vi "AnalysisConfig.vi"(8 "error in (no error)":errorcluster, 11 "AnalysisConfig":T6={"PortName"="WLAN_DUT0_ANT0", "PhyPort"=enum."Port5", "ExternalAtt"=0, "TriggerLevel"=-40, "NumberofChain"=1, "AcqLength"=0.0001, "MCSIndex"=7.0, "PhyType"=enum."OFDM", "Standard"=enum."802.11 n", "BW"=enum."20M", "TriggerSource"=enum."RIO0", "Freq"=5180000000.0, "LegacyDataRate"=enum."R1M", "PhyPort2"=enum."Port5", "Freq2"=5180000000.0, "ReferenceLevel(Peak)"=0.0}) -> (0 "error out":errorcluster, 3 "AnalysisConfigCMD":string[](array[string])=["MEMory:TABLe:DELete:ALL", "ROUTe:RFSG:PORT:DELete:ALL", "TRIG:RFSA:WLAN:EDGE RISING", "TRIG:RFSA:WLAN:MQTime  5e-6", "ROUTe:RFSA:PORT:DEFine 'wlan_DUT0_ant0','Port0'", "CONF:RFSA:WLAN:CSEG:EATT:ALL 0", "TRIG:RFSA:WLAN:SOUR 'RF0'", "TRIG:RFSA:WLAN:THR 0", "CONF:RFSA:WLAN:NCH 0", "CONF:RFSA:WLAN:CSEG:PORT \"wlan_DUT0_ant0\"", "CONF:RFSA:WLAN:CSEG:FREQ:CENT 5", "CONF:RFSA:WLAN:BWID 0", "CONF:RFSA:WLAN:STAN A", "CONF:RFSA:WLAN:ALENgth 0", "CONF:RFSA:WLAN:PACK:MCS 0", "CONF:RFSA:WLAN:PHY DSSS", "CONF:RFSA:WLAN:ACT:ALL 1", "CONF:RFSA:WLAN:CSEG:POW:AUTO ON", "CONF:RFSA:WLAN:PACK:NSTS 1 ", "CONF:RFSA:WLAN:PACK:GINT LONG", "CONF:RFSA:WLAN:PACK:DMOD ALL", "CONF:RFSA:WLAN:PACK:PAYL:LENGth 1500", "CONF:RFSA:WLAN:MEAS:MOD:ENAB ON", "CONF:RFSA:WLAN:MEAS:MOD:OFDM:EST:COFF ON", "CONF:RFSA:WLAN:MEAS:MOD:OFDM:EST:IMP ON", "CONF:RFSA:WLAN:MEAS:MOD:OFDM:TRAC:AMPL OFF", "CONF:RFSA:WLAN:MEAS:MOD:OFDM:TRAC:CHAN OFF", "CONF:RFSA:WLAN:MEAS:MOD:OFDM:TRAC:TIME ON", "CONF:RFSA:WLAN:MEAS:MOD:OFDM:TRAC:PHAS NONE", "CONF:RFSA:WLAN:MEAS:MOD:AVER:COUN 50", "CONF:RFSA:WLAN:MEAS:MOD:OFDM:MSYM 16", "CONF:RFSA:WLAN:MEAS:SEM:ENAB ON ", "CONF:RFSA:WLAN:MEAS:SEM:AVER:COUN 3", "CONF:RFSA:WLAN:MEAS:SEM:SPAN:AUTO:ENAB ON", "CONF:RFSA:WLAN:MEAS:OBW:ENAB ON", "CONF:RFSA:WLAN:MEAS:OBW:AVER:COUN 3", "CONF:RFSA:WLAN:MEAS:TXP:ENAB ON", "CONF:RFSA:WLAN:MEAS:TXP:AVER:COUN 3"])   [LabVIEW 2015]
uses:
  PhyPort.ctl
  PhyType.ctl
  standard.ctl
  BW.ctl
  LegacyDataRate.ctl
panel:
  out "size(s)":i32
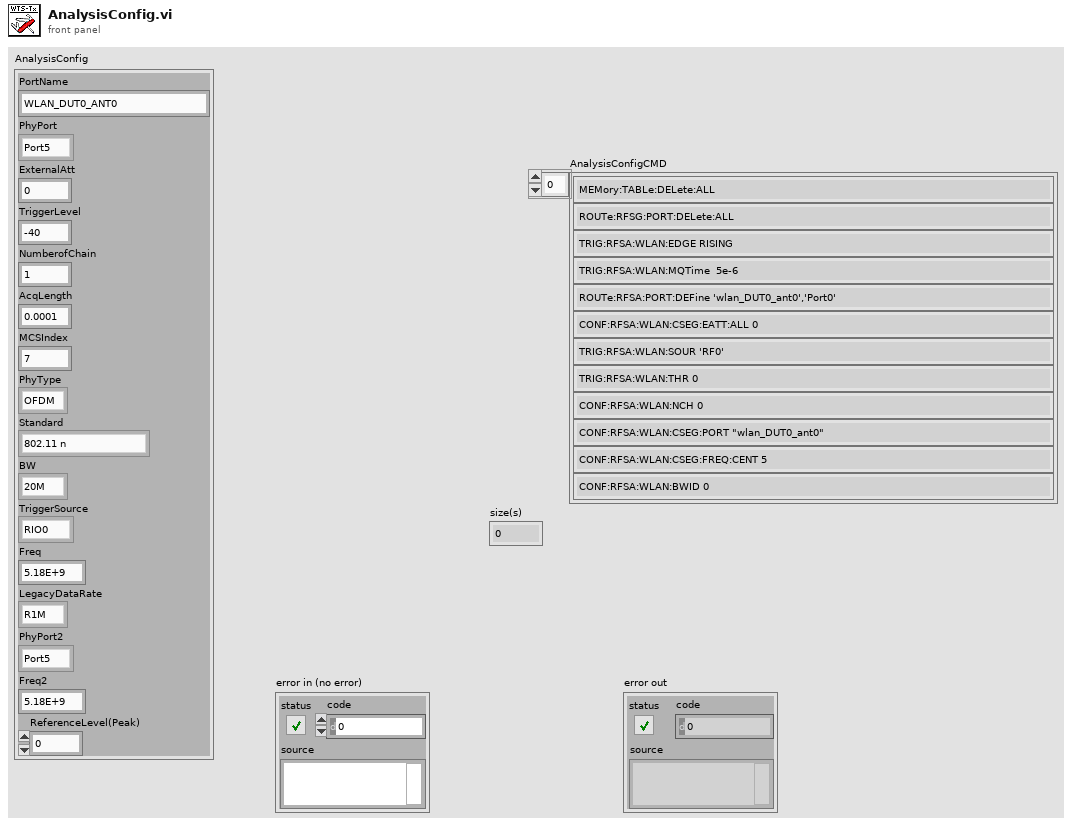
[diagram p1: front panel]
types:
  T1 = typedef "PhyPort.ctl" = enum16{"Port0", "Port1", "Port2", "Port3", "Port4", "Port5", "Port6", "Port7"}
  T2 = typedef "PhyType.ctl" = enum16{"DSSS", "OFDM", "HT", "VHT"}
  T3 = typedef "standard.ctl" = enum16{"802.11 a/g", "802.11 b/g", "802.11 g", "802.11 n", "802.11 ac"}
  T4 = typedef "BW.ctl" = enum16{"5M", "10M", "20M", "40M", "80M", "80P80M", "160M"}
  T5 = typedef "LegacyDataRate.ctl" = enum16{"R1M", "R2M", "R5M5", "R6M", "R9M", "R11M", "R12M", "R18M", "R24M", "R36M", "R48M", "R54M"}
  T6 = cluster{"PortName":string, "PhyPort":T1, "ExternalAtt":i32, "TriggerLevel":i32, "NumberofChain":i32, "AcqLength":dbl, "MCSIndex":dbl, "PhyType":T2, "Standard":T3, "BW":T4, "TriggerSource":enum16{"RIO0", "RIO1"}, "Freq":dbl, "LegacyDataRate":T5, "PhyPort2":T1, "Freq2":dbl, "ReferenceLevel(Peak)":dbl}
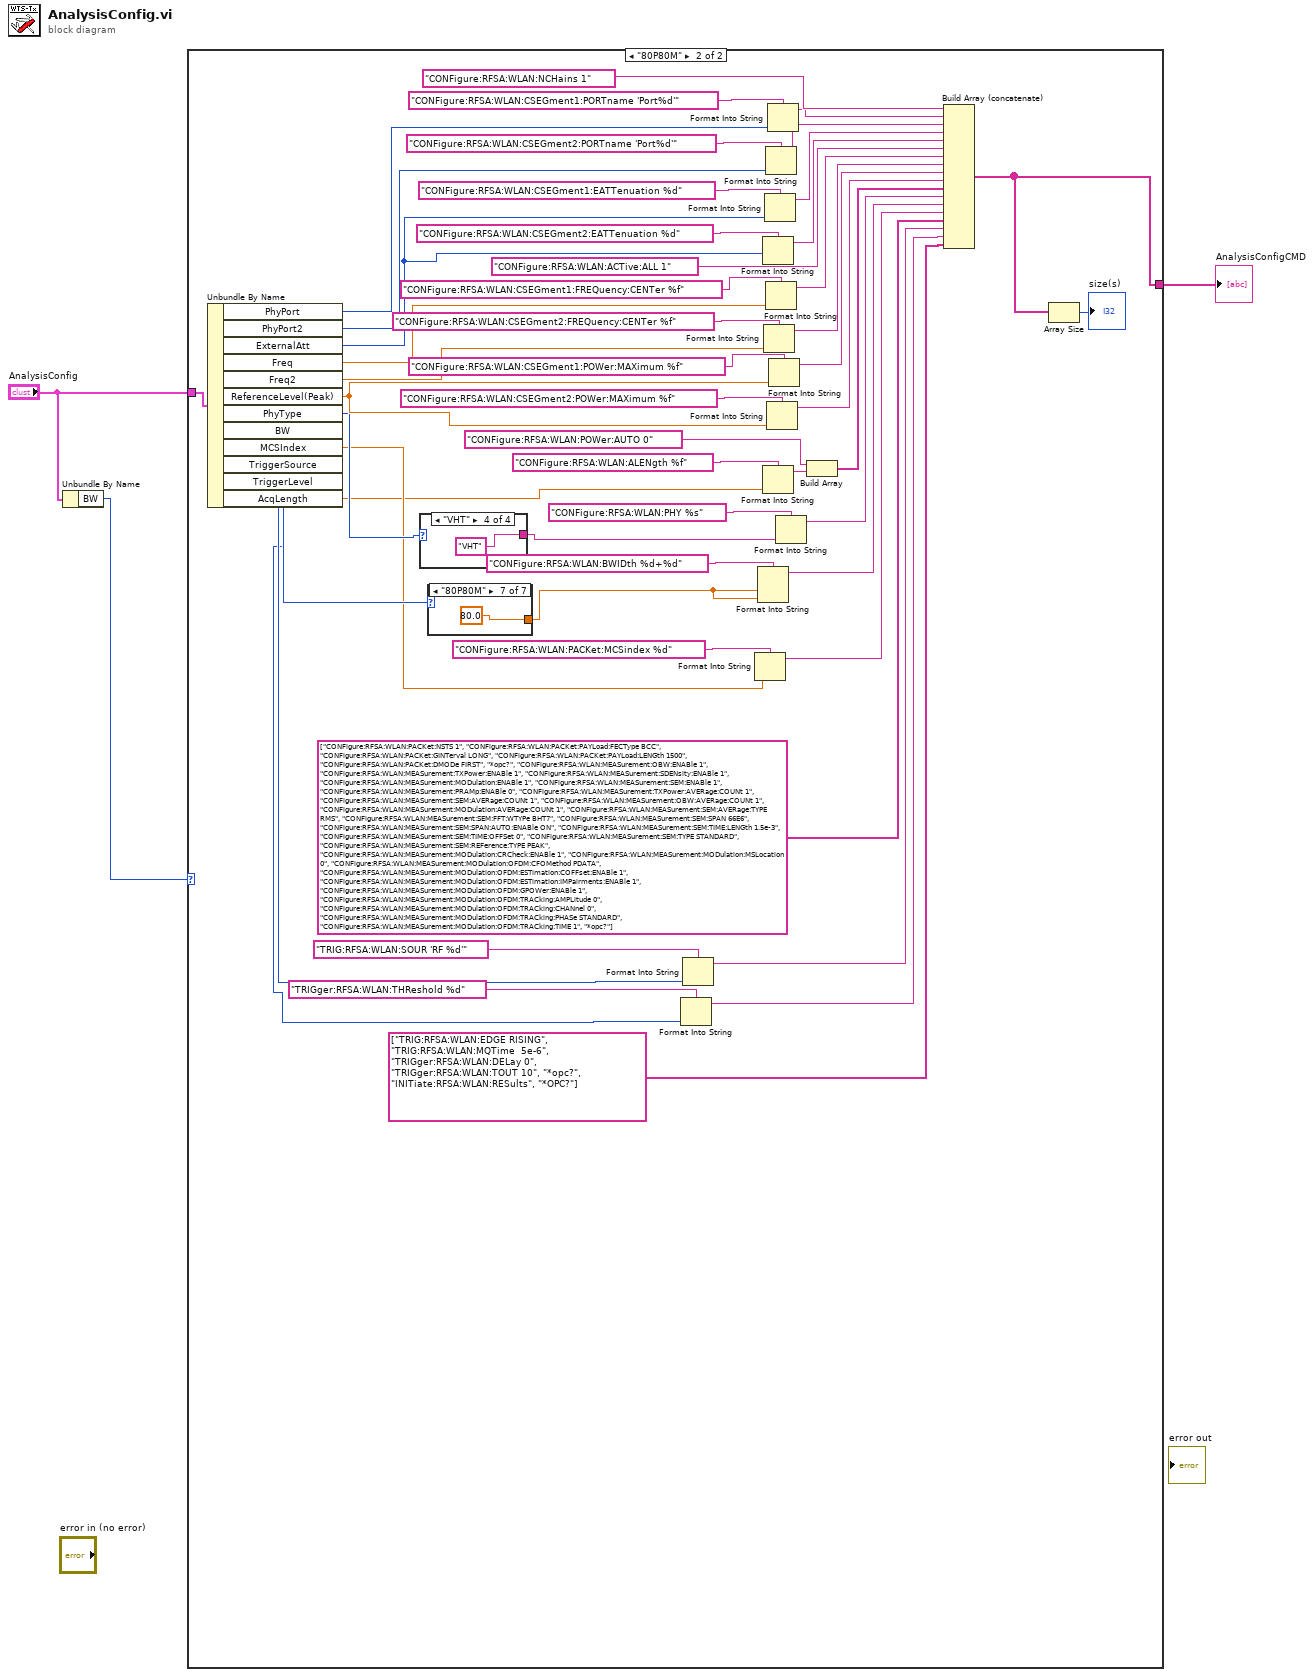
[diagram p0: block diagram]
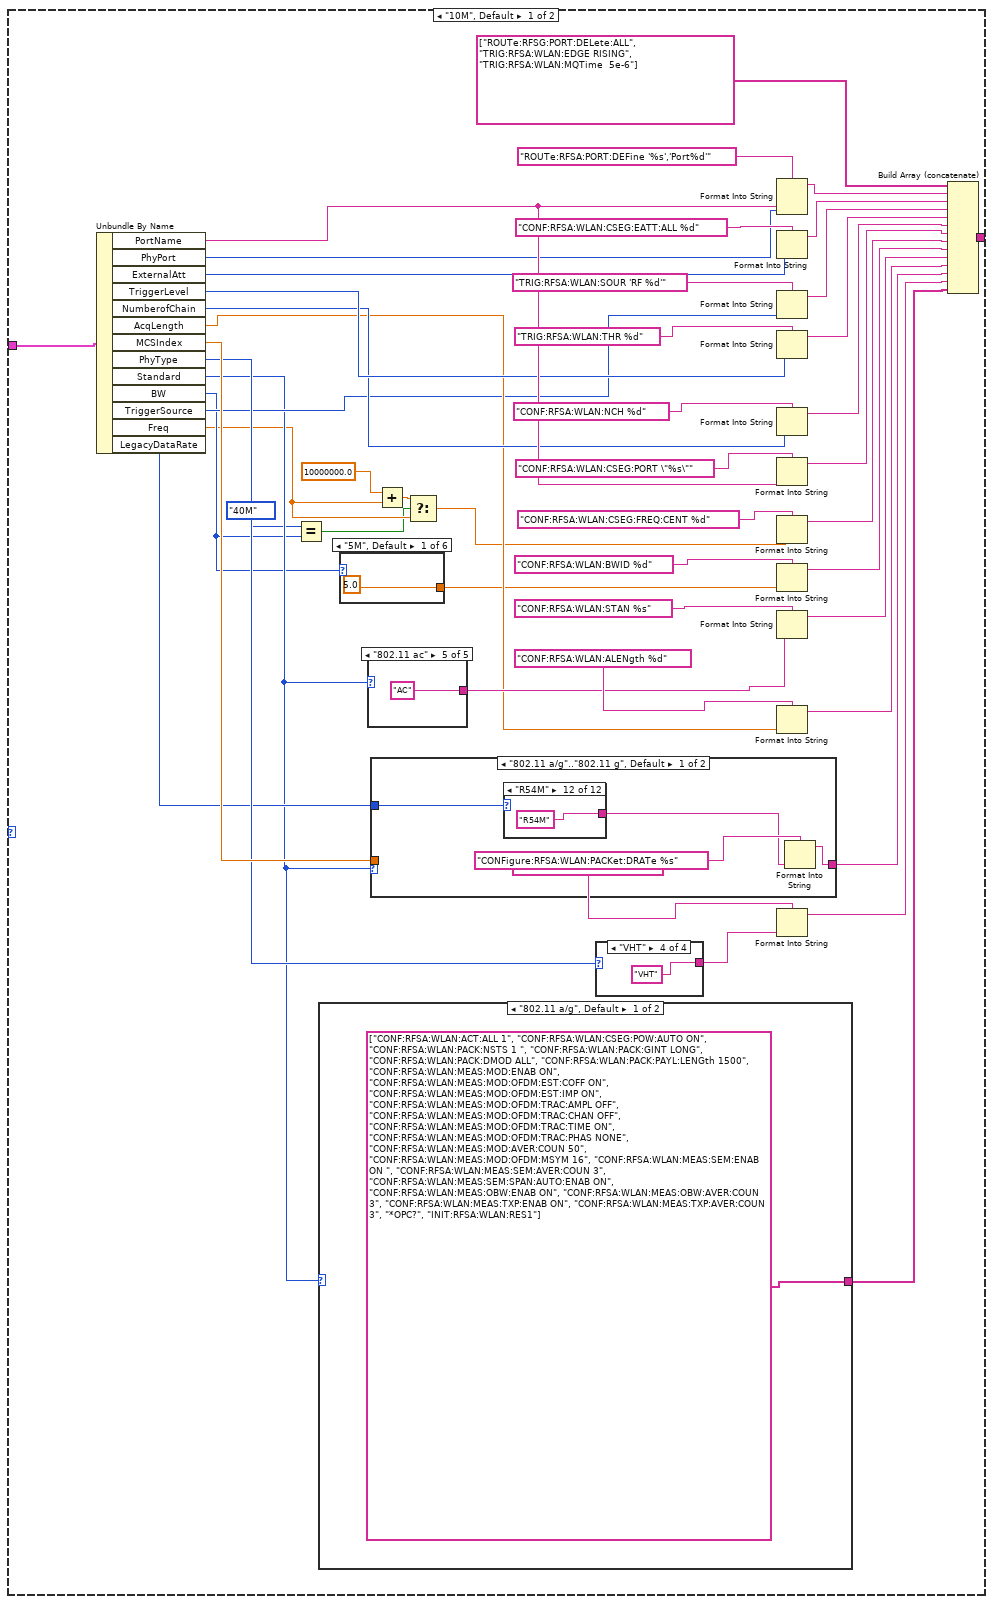
[diagram p2: hidden frame]
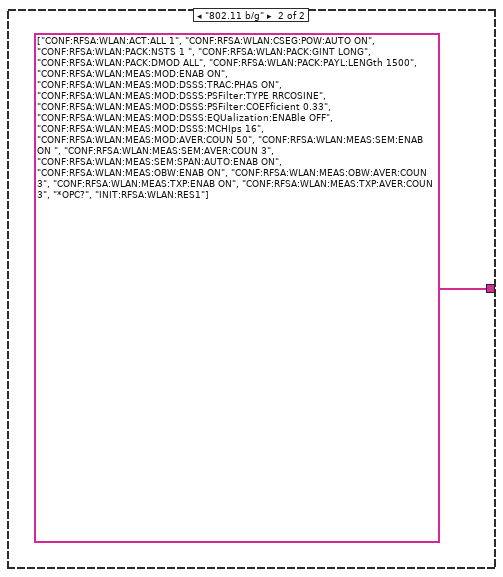
[diagram p3: hidden frame]
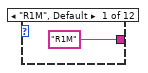
[diagram p4: hidden frame]
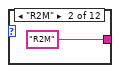
[diagram p5: hidden frame]
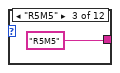
[diagram p6: hidden frame]
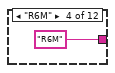
[diagram p7: hidden frame]
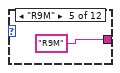
[diagram p8: hidden frame]
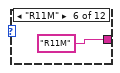
[diagram p9: hidden frame]
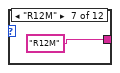
[diagram p10: hidden frame]
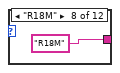
[diagram p11: hidden frame]
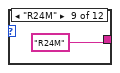
[diagram p12: hidden frame]
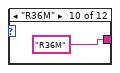
[diagram p13: hidden frame]
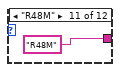
[diagram p14: hidden frame]
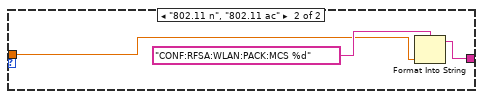
[diagram p15: hidden frame]
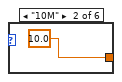
[diagram p16: hidden frame]
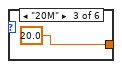
[diagram p17: hidden frame]
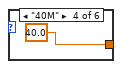
[diagram p18: hidden frame]
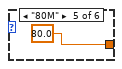
[diagram p19: hidden frame]
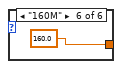
[diagram p20: hidden frame]
diagram:
  n1 = Unbundle By Name("AnalysisConfig") -> ("BW"=w1:T4)
  n2 = case shown="\"80P80M\"" w1 {
    tunnel: [w42 w89] -> w3
    tunnel: "AnalysisConfig" -> [w23 w137]
    frame "10M", Default {
      n3 = Unbundle By Name(w23) -> ("PortName"=w22:string, "PhyPort"=w21:T1, "ExternalAtt"=w20:i32, "TriggerLevel"=w19:i32, "NumberofChain"=w18:i32, "AcqLength"=w16:dbl, "MCSIndex"=w17:dbl, "PhyType"=w15:T2, "Standard"=w11:T3, "BW"=w10:T4, "TriggerSource"=w14:enum16{"RIO0", "RIO1"}, "Freq"=w7:dbl, "LegacyDataRate"=w12:T5)
      n4 = Equal?(x=BW."40M" ("BW"), y=w10) -> (x = y?=w4:bool)
      n5 = case shown="\"802.11 a/g\", Default" w11 {
        tunnel: [string[] ["CONF:RFSA:WLAN:ACT:ALL 1", "CONF:RFSA:WLAN:CSEG:POW:AUTO ON", "CONF:RFSA:WLAN:PACK:NSTS 1 ", "CONF:RFSA:WLAN:PACK:GINT LONG", "CONF:RFSA:WLAN:PACK:DMOD ALL", "CONF:RFSA:WLAN:PACK:PAYL:LENGth 1500", "CONF:RFSA:WLAN:MEAS:MOD:ENAB ON", "CONF:RFSA:WLAN:MEAS:MOD:OFDM:EST:COFF ON", "CONF:RFSA:WLAN:MEAS:MOD:OFDM:EST:IMP ON", "CONF:RFSA:WLAN:MEAS:MOD:OFDM:TRAC:AMPL OFF", "CONF:RFSA:WLAN:MEAS:MOD:OFDM:TRAC:CHAN OFF", "CONF:RFSA:WLAN:MEAS:MOD:OFDM:TRAC:TIME ON", "CONF:RFSA:WLAN:MEAS:MOD:OFDM:TRAC:PHAS NONE", "CONF:RFSA:WLAN:MEAS:MOD:AVER:COUN 50", "CONF:RFSA:WLAN:MEAS:MOD:OFDM:MSYM 16", "CONF:RFSA:WLAN:MEAS:SEM:ENAB ON ", "CONF:RFSA:WLAN:MEAS:SEM:AVER:COUN 3", "CONF:RFSA:WLAN:MEAS:SEM:SPAN:AUTO:ENAB ON", "CONF:RFSA:WLAN:MEAS:OBW:ENAB ON", "CONF:RFSA:WLAN:MEAS:OBW:AVER:COUN 3", "CONF:RFSA:WLAN:MEAS:TXP:ENAB ON", "CONF:RFSA:WLAN:MEAS:TXP:AVER:COUN 3", "*OPC?", "INIT:RFSA:WLAN:RES1"] string[] ["CONF:RFSA:WLAN:ACT:ALL 1", "CONF:RFSA:WLAN:CSEG:POW:AUTO ON", "CONF:RFSA:WLAN:PACK:NSTS 1 ", "CONF:RFSA:WLAN:PACK:GINT LONG", "CONF:RFSA:WLAN:PACK:DMOD ALL", "CONF:RFSA:WLAN:PACK:PAYL:LENGth 1500", "CONF:RFSA:WLAN:MEAS:MOD:ENAB ON", "CONF:RFSA:WLAN:MEAS:MOD:DSSS:TRAC:PHAS ON", "CONF:RFSA:WLAN:MEAS:MOD:DSSS:PSFilter:TYPE RRCOSINE", "CONF:RFSA:WLAN:MEAS:MOD:DSSS:PSFilter:COEFficient 0.33", "CONF:RFSA:WLAN:MEAS:MOD:DSSS:EQUalization:ENABle OFF", "CONF:RFSA:WLAN:MEAS:MOD:DSSS:MCHIps 16", "CONF:RFSA:WLAN:MEAS:MOD:AVER:COUN 50", "CONF:RFSA:WLAN:MEAS:SEM:ENAB ON ", "CONF:RFSA:WLAN:MEAS:SEM:AVER:COUN 3", "CONF:RFSA:WLAN:MEAS:SEM:SPAN:AUTO:ENAB ON", "CONF:RFSA:WLAN:MEAS:OBW:ENAB ON", "CONF:RFSA:WLAN:MEAS:OBW:AVER:COUN 3", "CONF:RFSA:WLAN:MEAS:TXP:ENAB ON", "CONF:RFSA:WLAN:MEAS:TXP:AVER:COUN 3", "*OPC?", "INIT:RFSA:WLAN:RES1"]] -> w25
        frame "802.11 a/g", Default {
        }
        frame "802.11 b/g" {
        }
      }
      n6 = case shown="\"5M\", Default" w10 {
        tunnel: [5.0 ("Freq") 10.0 ("Freq") 20.0 ("Freq") 40.0 ("Freq") 80.0 ("Freq") 160.0 ("Freq")] -> w13
        frame "5M", Default {
        }
        frame "10M" {
        }
        frame "20M" {
        }
        frame "40M" {
        }
        frame "80M" {
        }
        frame "160M" {
        }
      }
      n7 = case shown="\"802.11 ac\"" w11 {
        tunnel: ["A" ("Standard") "B" ("Standard") "G" ("Standard") "N" ("Standard") "AC" ("Standard")] -> w24
        frame "802.11 a/g", Default {
        }
        frame "802.11 b/g" {
        }
        frame "802.11 g" {
        }
        frame "802.11 n" {
        }
        frame "802.11 ac" {
        }
      }
      n8 = case shown="\"802.11 a/g\"..\"802.11 g\", Default" w11 {
        tunnel: [w54 w71] -> w27
        tunnel: w17 -> [_ w70]
        tunnel: w12 -> [w56 _]
        frame "802.11 a/g".."802.11 g", Default {
          n9 = case shown="\"R54M\"" w56 {
            tunnel: ["R1M" "R2M" "R5M5" "R6M" "R9M" "R11M" "R12M" "R18M" "R24M" "R36M" "R48M" "R54M"] -> w55
            frame "R1M", Default {
            }
            frame "R2M" {
            }
            frame "R5M5" {
            }
            frame "R6M" {
            }
            frame "R9M" {
            }
            frame "R11M" {
            }
            frame "R12M" {
            }
            frame "R18M" {
            }
            frame "R24M" {
            }
            frame "R36M" {
            }
            frame "R48M" {
            }
            frame "R54M" {
            }
          }
          n10 = Format Into String(format string="CONFigure:RFSA:WLAN:PACKet:DRATe %s", w55) -> (resulting string=w54:string)  [unwired: 2 in, 1 out]
        }
        frame "802.11 n", "802.11 ac" {
          n11 = Format Into String(format string="CONF:RFSA:WLAN:PACK:MCS %d", w70) -> (resulting string=w71:string)  [unwired: 2 in, 1 out]
        }
      }
      n12 = Add(x=10000000.0, y=w7) -> (x+y=w8:dbl)
      n13 = Select(t=w8, s=w4, f=w7) -> (s? t:f=w5:dbl)
      n14 = case shown="\"VHT\"" w15 {
        tunnel: ["DSSS" ("PhyType") "OFDM" ("PhyType") "HT" ("PhyType") "VHT" ("PhyType")] -> w34
        frame "DSSS", Default {
        }
        frame "OFDM" {
        }
        frame "HT" {
        }
        frame "VHT" {
        }
      }
      n15 = Format Into String(format string="ROUTe:RFSA:PORT:DEFine '%s','Port%d'", w22, w21) -> (resulting string=w46:string)  [unwired: 2 in, 1 out]
      n16 = Format Into String(format string="CONF:RFSA:WLAN:CSEG:EATT:ALL %d", w20) -> (resulting string=w45:string)  [unwired: 2 in, 1 out]
      n17 = Format Into String(format string="TRIG:RFSA:WLAN:SOUR 'RF %d'", w14) -> (resulting string=w44:string)  [unwired: 2 in, 1 out]
      n18 = Format Into String(format string="TRIG:RFSA:WLAN:THR %d", w19) -> (resulting string=w43:string)  [unwired: 2 in, 1 out]
      n19 = Format Into String(format string="CONF:RFSA:WLAN:NCH %d", w18) -> (resulting string=w33:string)  [unwired: 2 in, 1 out]
      n20 = Format Into String(format string="CONF:RFSA:WLAN:CSEG:PORT \"%s\"", w22) -> (resulting string=w32:string)  [unwired: 2 in, 1 out]
      n21 = Format Into String(format string="CONF:RFSA:WLAN:CSEG:FREQ:CENT %d", w5) -> (resulting string=w31:string)  [unwired: 2 in, 1 out]
      n22 = Format Into String(format string="CONF:RFSA:WLAN:BWID %d", w13) -> (resulting string=w30:string)  [unwired: 2 in, 1 out]
      n23 = Format Into String(format string="CONF:RFSA:WLAN:STAN %s", w24) -> (resulting string=w29:string)  [unwired: 2 in, 1 out]
      n24 = Format Into String(format string="CONF:RFSA:WLAN:ALENgth %d", w16) -> (resulting string=w28:string)  [unwired: 2 in, 1 out]
      n25 = Format Into String(format string="CONF:RFSA:WLAN:PHY %s", w34) -> (resulting string=w26:string)  [unwired: 2 in, 1 out]
      n26 = Build Array (concatenate)(string[] ["ROUTe:RFSG:PORT:DELete:ALL", "TRIG:RFSA:WLAN:EDGE RISING", "TRIG:RFSA:WLAN:MQTime  5e-6"], w46, w45, w44, w43, w33, w32, w31, w30, w29, w28, w27, w26, w25) -> (w42:string[])
    }
    frame "80P80M" {
      n27 = Unbundle By Name(w137) -> ("PhyPort"=w136:T1, "PhyPort2"=w135:T1, "ExternalAtt"=w128:i32, "Freq"=w122:dbl, "Freq2"=w121:dbl, "ReferenceLevel(Peak)"=w116:dbl, "PhyType"=w111:T2, "BW"=w108:T4, "MCSIndex"=w104:dbl, "TriggerSource"=w100:enum16{"RIO0", "RIO1"}, "TriggerLevel"=w98:i32, "AcqLength"=w93:dbl)
      n28 = case shown="\"VHT\"" w111 {
        tunnel: ["DSSS" ("PhyType") "OFDM" ("PhyType") "HT" ("PhyType") "VHT" ("PhyType")] -> w112
        frame "DSSS", Default {
        }
        frame "OFDM" {
        }
        frame "HT" {
        }
        frame "VHT" {
        }
      }
      n29 = case shown="\"80P80M\"" w108 {
        tunnel: [5.0 ("Freq") 10.0 ("Freq") 20.0 ("Freq") 40.0 ("Freq") 80.0 ("Freq") 160.0 ("Freq") 80.0] -> w107
        frame "5M", Default {
        }
        frame "10M" {
        }
        frame "20M" {
        }
        frame "40M" {
        }
        frame "80M" {
        }
        frame "160M" {
        }
        frame "80P80M" {
        }
      }
      n30 = Format Into String(format string="TRIGger:RFSA:WLAN:THReshold %d", w98) -> (resulting string=w96:string)  [unwired: 2 in, 1 out]
      n31 = Format Into String(format string="TRIG:RFSA:WLAN:SOUR 'RF %d'", w100) -> (resulting string=w97:string)  [unwired: 2 in, 1 out]
      n32 = Format Into String(format string="CONFigure:RFSA:WLAN:PACKet:MCSindex %d", w104) -> (resulting string=w103:string)  [unwired: 2 in, 1 out]
      n33 = Format Into String(format string="CONFigure:RFSA:WLAN:BWIDth %d+%d", w107, w107) -> (resulting string=w106:string)  [unwired: 2 in, 1 out]
      n34 = Format Into String(format string="CONFigure:RFSA:WLAN:CSEGment2:EATTenuation %d", w128) -> (resulting string=w126:string)  [unwired: 2 in, 1 out]
      n35 = Format Into String(format string="CONFigure:RFSA:WLAN:ALENgth %f", w93) -> (resulting string=w91:string)  [unwired: 2 in, 1 out]
      n36 = Format Into String(format string="CONFigure:RFSA:WLAN:CSEGment2:FREQuency:CENTer %f", w121) -> (resulting string=w119:string)  [unwired: 2 in, 1 out]
      n37 = Format Into String(format string="CONFigure:RFSA:WLAN:CSEGment1:EATTenuation %d", w128) -> (resulting string=w127:string)  [unwired: 2 in, 1 out]
      n38 = Format Into String(format string="CONFigure:RFSA:WLAN:CSEGment2:PORTname 'Port%d'", w135) -> (resulting string=w131:string)  [unwired: 2 in, 1 out]
      n39 = Format Into String(format string="CONFigure:RFSA:WLAN:CSEGment1:FREQuency:CENTer %f", w122) -> (resulting string=w120:string)  [unwired: 2 in, 1 out]
      n40 = Format Into String(format string="CONFigure:RFSA:WLAN:CSEGment2:POWer:MAXimum %f", w116) -> (resulting string=w114:string)  [unwired: 2 in, 1 out]
      n41 = Format Into String(format string="CONFigure:RFSA:WLAN:CSEGment1:PORTname 'Port%d'", w136) -> (resulting string=w132:string)  [unwired: 2 in, 1 out]
      n42 = Format Into String(format string="CONFigure:RFSA:WLAN:CSEGment1:POWer:MAXimum %f", w116) -> (resulting string=w115:string)  [unwired: 2 in, 1 out]
      n43 = Format Into String(format string="CONFigure:RFSA:WLAN:PHY %s", w112) -> (resulting string=w110:string)  [unwired: 2 in, 1 out]
      n44 = Build Array("CONFigure:RFSA:WLAN:POWer:AUTO 0", w91) -> (w90:string[])
      n45 = Build Array (concatenate)("CONFigure:RFSA:WLAN:NCHains 1", w132, w131, w127, w126, "CONFigure:RFSA:WLAN:ACTive:ALL 1" ("format string"), w120, w119, w115, w114, w90, w110, w106, w103, string[] ["CONFigure:RFSA:WLAN:PACKet:NSTS 1", "CONFigure:RFSA:WLAN:PACKet:PAYLoad:FECType BCC", "CONFigure:RFSA:WLAN:PACKet:GINTerval LONG", "CONFigure:RFSA:WLAN:PACKet:PAYLoad:LENGth 1500", "CONFigure:RFSA:WLAN:PACKet:DMODe FIRST", "*opc?", "CONFigure:RFSA:WLAN:MEASurement:OBW:ENABle 1", "CONFigure:RFSA:WLAN:MEASurement:TXPower:ENABle 1", "CONFigure:RFSA:WLAN:MEASurement:SDENsity:ENABle 1", "CONFigure:RFSA:WLAN:MEASurement:MODulation:ENABle 1", "CONFigure:RFSA:WLAN:MEASurement:SEM:ENABle 1", "CONFigure:RFSA:WLAN:MEASurement:PRAMp:ENABle 0", "CONFigure:RFSA:WLAN:MEASurement:TXPower:AVERage:COUNt 1", "CONFigure:RFSA:WLAN:MEASurement:SEM:AVERage:COUNt 1", "CONFigure:RFSA:WLAN:MEASurement:OBW:AVERage:COUNt 1", "CONFigure:RFSA:WLAN:MEASurement:MODulation:AVERage:COUNt 1", "CONFigure:RFSA:WLAN:MEASurement:SEM:AVERage:TYPE RMS", "CONFigure:RFSA:WLAN:MEASurement:SEM:FFT:WTYPe BHT7", "CONFigure:RFSA:WLAN:MEASurement:SEM:SPAN 66E6", "CONFigure:RFSA:WLAN:MEASurement:SEM:SPAN:AUTO:ENABle ON", "CONFigure:RFSA:WLAN:MEASurement:SEM:TIME:LENGth 1.5e-3", "CONFigure:RFSA:WLAN:MEASurement:SEM:TIME:OFFSet 0", "CONFigure:RFSA:WLAN:MEASurement:SEM:TYPE STANDARD", "CONFigure:RFSA:WLAN:MEASurement:SEM:REFerence:TYPE PEAK", "CONFigure:RFSA:WLAN:MEASurement:MODulation:CRCheck:ENABle 1", "CONFigure:RFSA:WLAN:MEASurement:MODulation:MSLocation 0", "CONFigure:RFSA:WLAN:MEASurement:MODulation:OFDM:CFOMethod PDATA", "CONFigure:RFSA:WLAN:MEASurement:MODulation:OFDM:ESTimation:COFFset:ENABle 1", "CONFigure:RFSA:WLAN:MEASurement:MODulation:OFDM:ESTimation:IMPairments:ENABle 1", "CONFigure:RFSA:WLAN:MEASurement:MODulation:OFDM:GPOWer:ENABle 1", "CONFigure:RFSA:WLAN:MEASurement:MODulation:OFDM:TRACking:AMPLitude 0", "CONFigure:RFSA:WLAN:MEASurement:MODulation:OFDM:TRACking:CHANnel 0", "CONFigure:RFSA:WLAN:MEASurement:MODulation:OFDM:TRACking:PHASe STANDARD", "CONFigure:RFSA:WLAN:MEASurement:MODulation:OFDM:TRACking:TIME 1", "*opc?"], w97, w96, string[] ["TRIG:RFSA:WLAN:EDGE RISING", "TRIG:RFSA:WLAN:MQTime  5e-6", "TRIGger:RFSA:WLAN:DELay 0", "TRIGger:RFSA:WLAN:TOUT 10", "*opc?", "INITiate:RFSA:WLAN:RESults", "*OPC?"]) -> (w89:string[])
      n46 = Array Size(array=w89) -> (size(s)=→"size(s)":i32)
    }
  }
  "AnalysisConfigCMD" <- w3
